vi "Get All Subscibers.vi"(8 "error in (no error)":errorcluster, 11 "Topic Actor in":refnum<class "Topic Actor.lvclass">) -> (0 "error out":errorcluster, 2 "Subscribers":refnum<class "Message Transport Interface.lvclass">[](array[class]), 3 "Topic Actor out":refnum<class "Topic Actor.lvclass">)   [LabVIEW 2016, in "Stream Mediator.lvlib" / "Topic Actor.lvclass"]
uses:
  <userlib>/Composed Systems/Stream/Mediator/Classes/Topic Actor/Topic Actor.lvclass
  <userlib>/Composed Systems/Stream/Mediator/Classes/Message Transport Interface/Message Transport Interface.lvclass
  <userlib>/Composed Systems/Stream/Mediator/Classes/Topic Actor/Topic Actor.lvclass/Topic Actor.ctl
  <userlib>/Composed Systems/Stream/Mediator/Classes/Subscriber Look Up Table/Subscriber Look Up Table.lvclass
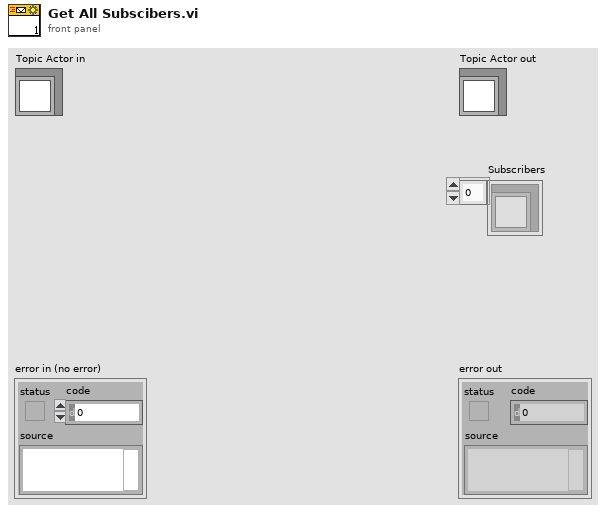
[diagram p1: front panel]
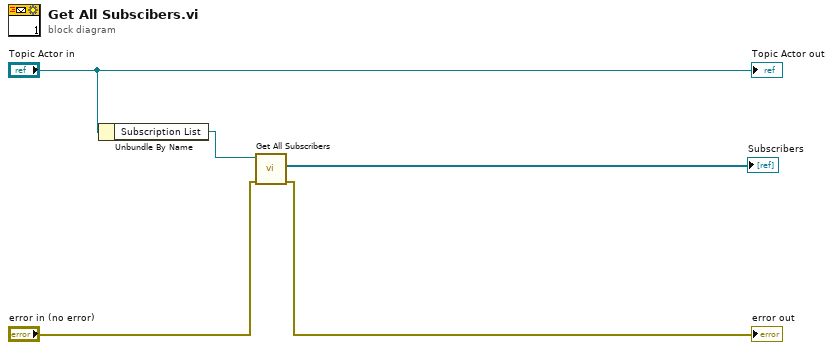
[diagram p0: block diagram]
diagram:
  n1 = Unbundle By Name("Topic Actor in") -> ("Subscription List"=w4:refnum<class "Subscriber Look Up Table.lvclass">)
  n2 = call <userlib>:"Get All Subscribers.vi"("error in (no error)"="error in (no error)", "Subscriber Look Up Table in"=w4) -> ("error out"=→"error out":errorcluster, "Subscribers"=→"Subscribers":refnum<class "Message Transport Interface.lvclass">[])  [unwired: 7 in, 1 out]
  "Topic Actor out" <- "Topic Actor in"
